vi "Error Query.vi"(8 "error in (no error)":errorcluster, 11 "VISA resource name":refnum<visa-resource-name>) -> (0 "error out":errorcluster, 1 "Error Message":string, 2 "Error Code":i32[](array[numeric]), 3 "VISA resource name out":refnum<visa-resource-name>)   [LabVIEW 2021, in "Yokogawa WT1800 Series.lvlib"]
doc: "Queries the instrument for any errors in the instrument's error queue. It will continue to read errors until all errors have been read from the instrument. Any errors will be returned in the Error Out cluster.\n\n<b>Note:</b>\nThis VI is called automatically by most driver VIs so it is not usually necessary to call this in an application."
uses:
  <instrlib>/Yokogawa WT1800 Series/Yokogawa WT1800 Series.lvlib
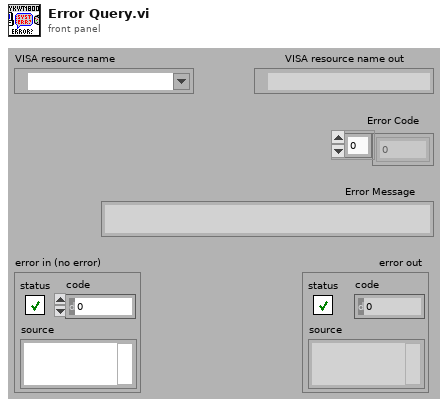
[diagram p1: front panel]
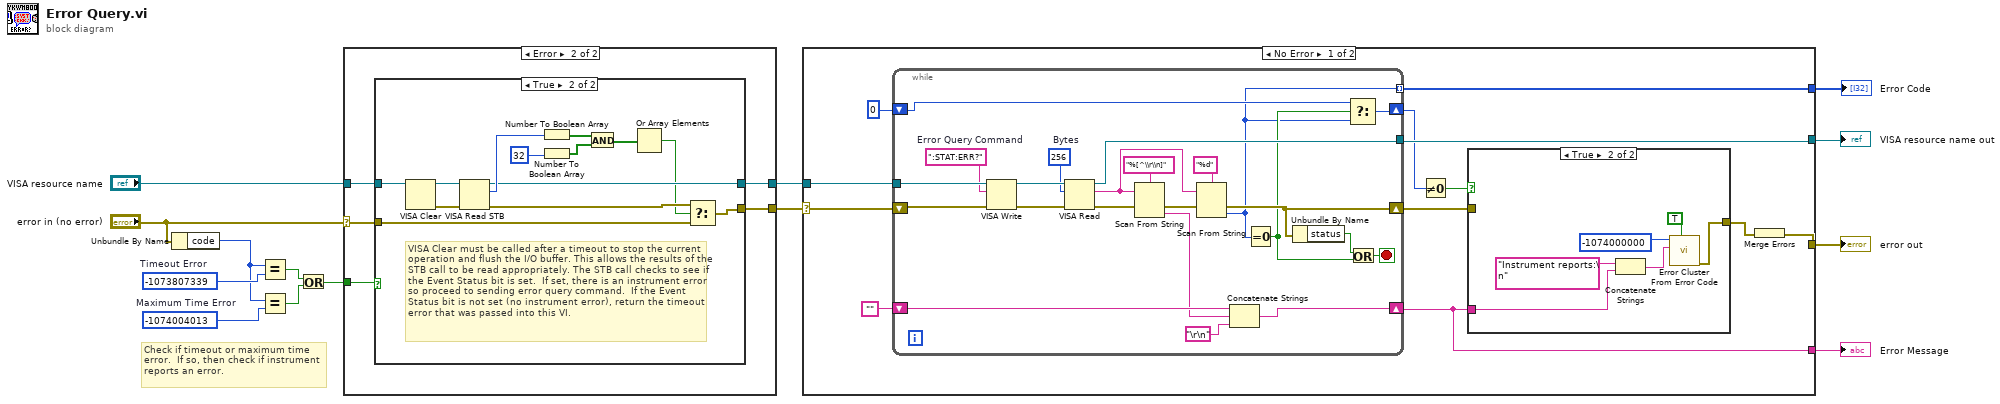
[diagram p0: block diagram]
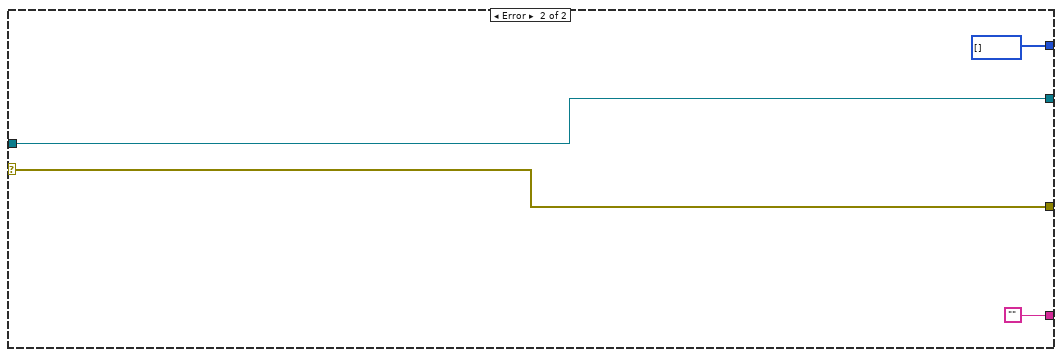
[diagram p5: hidden frame]
diagram:
  w1 = -1074004013  # Maximum Time Error
  w12 = -1073807339  # Timeout Error
  # "Check if timeout or maximum time error.  If so, then check if instrument reports an error."
  n1 = Unbundle By Name("error in (no error)") -> ("code"=w2:i32)
  n2 = Equal?(x=w2, y=w12) -> (x = y?=w9:bool)
  n3 = Equal?(x=w2, y=w1) -> (x = y?=w3:bool)
  n4 = Or(x=w9, y=w3) -> (x .or. y?=w4:bool)
  n5 = case shown="Error" "error in (no error)" {
    selector: "error in (no error)" -> [w15 w19]
    tunnel: "VISA resource name" -> [w16 w21]
    tunnel: [w16 w20] -> w6
    tunnel: [w15 w18] -> w5
    tunnel: w4 -> [_ w17]
    frame No Error {
    }
    frame Error {
      n6 = case shown="True" w17 {
        tunnel: w21 -> [w23 w33]
        tunnel: [w23 w28] -> w20
        tunnel: w19 -> [w22 w25]
        tunnel: [w22 w26] -> w18
        frame False {
          # "Error code not a timeout, so best to pass on to"
        }
        frame True {
          # "VISA Clear must be called after a timeout to stop the current operation and flush the I/O buffer. This allows the results of the  STB call to be read appropriately. The STB call checks to see if the Event Status bit is set.  If set, there is an instrument error so proceed to sending error query command.  If the Event Status bit is not set (no instrument error), return the timeout error that was passed into this VI."
          n7 = VISA Clear(VISA resource name=w33) -> (VISA resource name out=w35:refnum<visa-resource-name>, error out=w36:errorcluster)  [unwired: 1 in]
          n8 = VISA Read STB(8:w36, 11:w35) -> (0:w27:errorcluster, 2:w32:u16, 3:w28:refnum<visa-resource-name>)
          n9 = Number To Boolean Array(number=w32) -> (Boolean array=w31:bool[])
          n10 = Number To Boolean Array(number=u32 32 ("l")) -> (Boolean array=w30:bool[])
          n11 = And(x=w31, y=w30) -> (x .and. y?=w29:bool[])
          n12 = Or Array Elements(Boolean array=w29) -> (logical OR=w24:bool)
          n13 = Select(t=w27, s=w24, f=w25) -> (s? t:f=w26:errorcluster)
        }
      }
    }
  }
  n14 = case shown="No Error" w5 {
    selector: w5 -> [w37 w79]
    tunnel: [w48 w82] -> w14
    tunnel: w6 -> [w47 w82]
    tunnel: [w45 w79] -> w13
    tunnel: [w41 ""] -> w11
    tunnel: [w40 i32[] []] -> w10
    frame No Error {
      n15 = while {
        tunnel: [w78] -> w48
        tunnel: w47 -> [w77]
        shift-right: [w66] -> w41
        shift-left: "" -> [w69]
        shift-right: [w64] -> w42
        shift-left: 0 -> [w65]
        shift-right: [w62] -> w39
        shift-left: w37 -> [w63]
        tunnel: [w57] -> w40 mode=indexing
        stop <- w71 stop-if-true
        w75 = u32 256  # Bytes
        w73 = ":STAT:ERR?"  # Error Query Command
        n16 = VISA Write(VISA resource name=w77, write buffer=w73, error in (no error)=w63) -> (VISA resource name out=w76:refnum<visa-resource-name>, error out=w74:errorcluster)  [unwired: 1 out]
        n17 = VISA Read(VISA resource name=w76, byte count=w75, error in (no error)=w74) -> (VISA resource name out=w78:refnum<visa-resource-name>, read buffer=w56:string, error out=w61:errorcluster)  [unwired: 1 out]
        n18 = Scan From String(format string="%[^\\r\\n]", input string=w56, error in=w61) -> (error out=w60:errorcluster, output 1=w67:string)  [unwired: 2 in, 2 out]
        n19 = Scan From String(format string="%d", input string=w56, error in=w60) -> (error out=w62:errorcluster, output 1=w57:i32)  [unwired: 2 in, 2 out]
        n20 = Concatenate Strings(w69, w67, "\r\n") -> (w66:string)
        n21 = Equal To 0?(x=w57) -> (x = 0?=w58:bool)
        n22 = Unbundle By Name(w62) -> ("status"=w59:bool)
        n23 = Select(t=w65, s=w58, f=w57) -> (s? t:f=w64:i32)
        n24 = Or(x=w59, y=w58) -> (x .or. y?=w71:bool)
      }
      n25 = Not Equal To 0?(x=w42) -> (x != 0?=w43:bool)
      n26 = case shown="True" w43 {
        tunnel: w41 -> [_ w54]
        tunnel: [w49 w50] -> w38
        tunnel: w39 -> [w49 _]
        frame False {
        }
        frame True {
          n27 = Concatenate Strings("Instrument reports:\n" ("Source"), w54) -> (w51:string)
          n28 = call <vilib>:"Error Cluster From Error Code.vi"("show call chain? (False)"=TRUE, "error message (\"\")"=w51, "error code (0)"=-1074000000 ("Code")) -> ("error out"=w50:errorcluster)  [unwired: 6 in]
        }
      }
      n29 = Merge Errors(w38) -> (w45:errorcluster)
    }
    frame Error {
    }
  }
  "VISA resource name out" <- w14
  "error out" <- w13
  "Error Message" <- w11
  "Error Code" <- w10
